vi "RhodeAndSchwartz-forSweepESR.vi"(0 "Ring":u16(ring)=1 items=["FREQSET", "SWEEP", "RF OFF", "ABORT"], 1 "Start frequency":dbl=1.0, 2 "Stop frequency":dbl=2.0, 3 "Steps":i32=2, 4 "UNIT":u16(ring)=1 items=["GHz", "MHz"], 5 "VISA resource name":refnum<visa-resource-name>="GPIB0::28::INSTR", 6 "Power level (dBm)":dbl, 7 "Frequency":dbl=2.0) -> ()   [LabVIEW 2010]
panel:
  # "CW"
  # "Created by Nusran. Sep 2014"
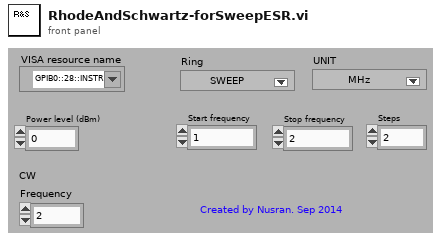
[diagram p1: front panel]
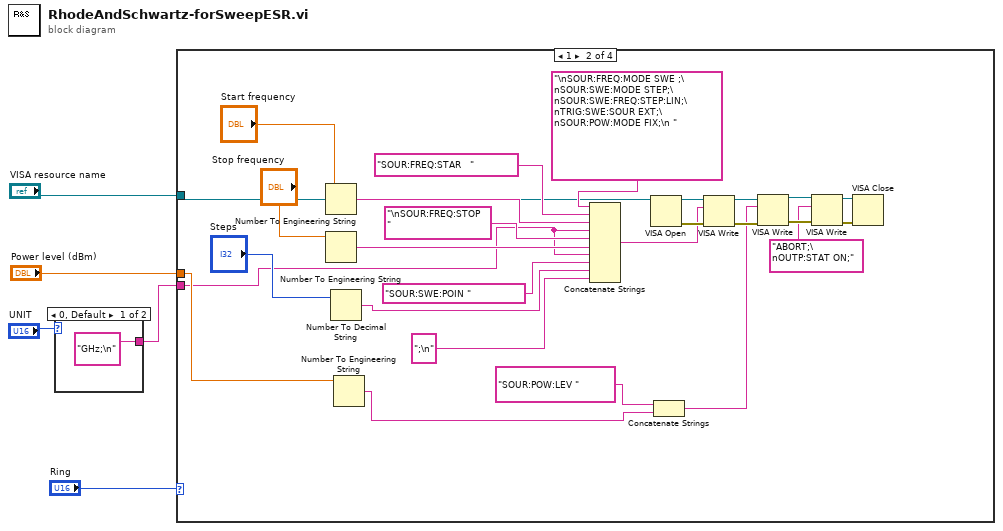
[diagram p0: block diagram]
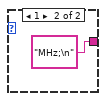
[diagram p2: hidden frame]
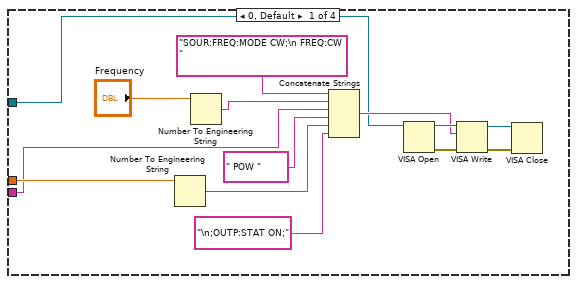
[diagram p3: hidden frame]
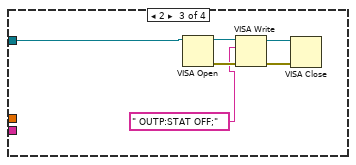
[diagram p4: hidden frame]
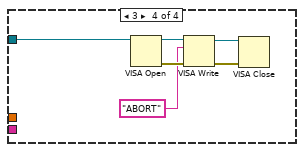
[diagram p5: hidden frame]
diagram:
  n1 = case shown="0, Default" "UNIT" {
    tunnel: ["GHz;\n" ("string") "MHz;\n" ("string")] -> w1
    frame 0, Default {
    }
    frame 1 {
    }
  }
  n2 = case shown="1" "Ring" {
    tunnel: "Power level (dBm)" -> [w10 w31 _ _]
    tunnel: "VISA resource name" -> [w9 w34 w50 w55]
    tunnel: w1 -> [w8 w22 _ _]
    frame 0, Default {
      n3 = Number To Engineering String(4:w10) -> (0:w13:string)  [unwired: 3 in]
      n4 = Number To Engineering String(4:"Frequency") -> (0:w15:string)  [unwired: 3 in]
      n5 = Concatenate Strings("SOUR:FREQ:MODE CW;\n FREQ:CW " ("string"), w15, w8, " POW " ("string"), w13, "\n;OUTP:STAT ON;" ("string")) -> (w11:string)
      n6 = VISA Open(VISA resource name=w9) -> (VISA resource name=w21:refnum<visa-resource-name>, error out=w18:errorcluster)  [unwired: 4 in]
      n7 = VISA Write(VISA resource name=w21, write buffer=w11, error in (no error)=w18) -> (VISA resource name out=w19:refnum<visa-resource-name>, error out=w20:errorcluster)  [unwired: 1 out]
      n8 = VISA Close(VISA resource name=w19, error in (no error)=w20) -> ()  [unwired: 1 out]
    }
    frame 1 {
      n9 = Number To Engineering String(4:"Start frequency") -> (0:w45:string)  [unwired: 3 in]
      n10 = Number To Engineering String(4:"Stop frequency") -> (0:w43:string)  [unwired: 3 in]
      n11 = Number To Decimal String(number="Steps") -> (decimal integer string=w36:string)  [unwired: 1 in]
      n12 = Number To Engineering String(4:w31) -> (0:w30:string)  [unwired: 3 in]
      n13 = Concatenate Strings("\nSOUR:FREQ:MODE SWE ;\nSOUR:SWE:MODE STEP;\nSOUR:SWE:FREQ:STEP:LIN;\nTRIG:SWE:SOUR EXT;\nSOUR:POW:MODE FIX;\n " ("string"), "SOUR:FREQ:STAR   " ("string"), w45, w22, "\nSOUR:FREQ:STOP  " ("string"), w43, w22, "SOUR:SWE:POIN " ("string"), w36, ";\n" ("string")) -> (w46:string)
      n14 = VISA Open(VISA resource name=w34) -> (VISA resource name=w48:refnum<visa-resource-name>, error out=w47:errorcluster)  [unwired: 4 in]
      n15 = Concatenate Strings("SOUR:POW:LEV " ("string"), w30) -> (w28:string)
      n16 = VISA Write(VISA resource name=w48, write buffer=w46, error in (no error)=w47) -> (VISA resource name out=w33:refnum<visa-resource-name>, error out=w32:errorcluster)  [unwired: 1 out]
      n17 = VISA Write(VISA resource name=w33, write buffer=w28, error in (no error)=w32) -> (VISA resource name out=w27:refnum<visa-resource-name>, error out=w26:errorcluster)  [unwired: 1 out]
      n18 = VISA Write(VISA resource name=w27, write buffer="ABORT;\nOUTP:STAT ON;" ("string"), error in (no error)=w26) -> (VISA resource name out=w25:refnum<visa-resource-name>, error out=w24:errorcluster)  [unwired: 1 out]
      n19 = VISA Close(VISA resource name=w25, error in (no error)=w24) -> ()  [unwired: 1 out]
    }
    frame 2 {
      n20 = VISA Open(VISA resource name=w50) -> (VISA resource name=w54:refnum<visa-resource-name>, error out=w51:errorcluster)  [unwired: 4 in]
      n21 = VISA Write(VISA resource name=w54, write buffer=" OUTP:STAT OFF;" ("string"), error in (no error)=w51) -> (VISA resource name out=w52:refnum<visa-resource-name>, error out=w53:errorcluster)  [unwired: 1 out]
      n22 = VISA Close(VISA resource name=w52, error in (no error)=w53) -> ()  [unwired: 1 out]
    }
    frame 3 {
      n23 = VISA Open(VISA resource name=w55) -> (VISA resource name=w60:refnum<visa-resource-name>, error out=w57:errorcluster)  [unwired: 4 in]
      n24 = VISA Write(VISA resource name=w60, write buffer="ABORT" ("string"), error in (no error)=w57) -> (VISA resource name out=w58:refnum<visa-resource-name>, error out=w59:errorcluster)  [unwired: 1 out]
      n25 = VISA Close(VISA resource name=w58, error in (no error)=w59) -> ()  [unwired: 1 out]
    }
  }
